vi "Line Configuration Dialog.vi"(8 "error in":errorcluster, 9 "engine configuration in":refnum<class "engine configuration.lvclass">, 10 "dds configuration":refnum<class "dds configuration.lvclass">, 11 "Line":T5) -> (0 "error out":errorcluster, 1 "success":bool, 2 "changed":bool, 3 "Mappings out":T4)   [LabVIEW 2020, in "DDS editor node.lvclass"]
uses:
  dds editor node.lvclass
  module/configuration/Line.ctl
  <vilib>/NI/Tag Bus Module Framework/channel/TBM channel.lvclass
  C:/Program Files (x86)/National Instruments/LabVIEW 2020/vi.lib/NI/Tag Bus/tag/tag descriptor.lvclass
  <vilib>/RTI DDS Toolkit/Types/RTI DDS Advanced Reader Configuration.ctl
  Mappings.ctl
  Map.ctl
  permissions.ctl
  <vilib>/NI/Module Execution Interface/Engine Configuration/engine configuration.lvclass
  module/configuration/dds configuration.lvclass
  C:/Program Files (x86)/National Instruments/LabVIEW 2020/vi.lib/NI/Configuration Framework/serializable configuration/NISE_CEF_serializable configuration.lvclass
  <vilib>/NI/Tag Bus Module Framework/channel/TBM channel.lvclass/TBM channel.ctl
  <vilib>/NI/Tag Bus/tag/tag descriptor.lvclass/tag descriptor.ctl
  <vilib>/NI/Configuration Framework/serializable configuration/NISE_CEF_serializable configuration.lvclass/NISE_CEF_serializable configuration.ctl
  <vilib>/NI/Tag Bus/tag/write tag name.vi
  <vilib>/NI/Tag Bus/tag/write data type.vi
  <vilib>/NI/Tag Bus Module Framework/channel/Write channel classification.vi
  <vilib>/NI/Tag Bus Module Framework/channel/Read channel classification.vi
  <vilib>/NI/Tag Bus/tag/read data type.vi
  <vilib>/NI/Configuration Framework/serializable configuration/Read UID.vi
  <vilib>/Utility/LVClass/Get LV Class Name.vi
  <vilib>/NI/Configuration Framework/error generator/NISE_error generator.vi
  <vilib>/NI/Tag Bus/tag/tag descriptor.lvclass
  <vilib>/RTI DDS Toolkit/Library/LVDDS_library.lvlib
panel:
  in  "Reader Configuration":T1={"typeName"="", "keyName"="", "domainParticipantQoSProfile"="", "dataReaderQoSProfile"="LabVIEWLibrary::DefaultProfile", "forceArrayMapping?"=FALSE, "forceExclusiveReader?"=FALSE, "forceRead? (only ExclusiveReader)"=FALSE, "forceUnboundedString?"=FALSE}
  in  "Domain ID":u32
  in  "Writer Configuration":T2={"typeName"="", "keyName"="", "domainParticipantQoSProfile"="", "dataWriterQoSProfile"="LabVIEWLibrary::DefaultProfile", "forceArrayMapping?"=FALSE, "forceUnboundedString?"=FALSE}
  out "errors":string
  in  "Access Type":T3
  in  "Mapped Tag":i32(listbox)
  in  "Data Type":i32(listbox)
  in  "Topic Name":string
  in  "cancel":bool
  in  "ok":bool
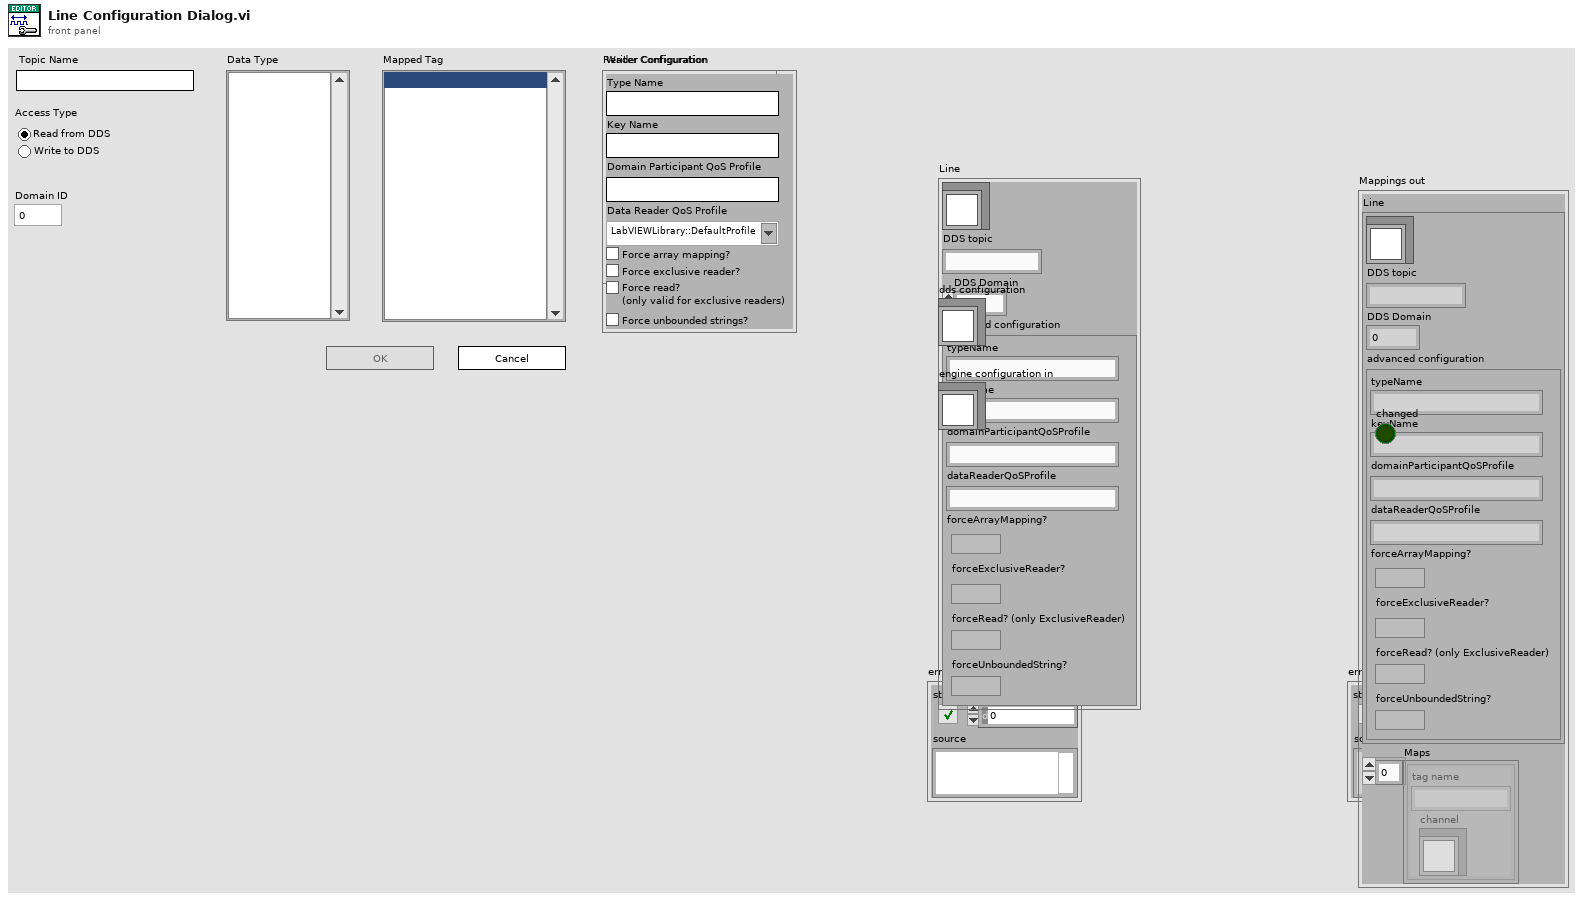
[diagram p1: front panel]
types:
  T1 = cluster{"typeName":string, "keyName":string, "domainParticipantQoSProfile":string, "dataReaderQoSProfile":string, "forceArrayMapping?":bool, "forceExclusiveReader?":bool, "forceRead? (only ExclusiveReader)":bool, "forceUnboundedString?":bool}
  T2 = cluster{"typeName":string, "keyName":string, "domainParticipantQoSProfile":string, "dataWriterQoSProfile":string, "forceArrayMapping?":bool, "forceUnboundedString?":bool}
  T3 = typedef "DDS editor node.lvclass/permissions.ctl" = enum32{"Read from DDS", "Write to DDS"}
  T4 = typedef "DDS editor node.lvclass/Mappings.ctl" = cluster{"Line":T5, "Maps":T7[]}
  T5 = typedef "DDS configuration.lvclass/Line.ctl" = cluster{"channel":refnum<class "TBM channel.lvclass">, "DDS topic":string, "DDS Domain":u32, "advanced configuration":T6}
  T6 = typedef "LVDDS_library.lvlib/RTI DDS Advanced Reader Configuration.ctl" = cluster{"typeName":string, "keyName":string, "domainParticipantQoSProfile":string, "dataReaderQoSProfile":string, "forceArrayMapping?":bool, "forceExclusiveReader?":bool, "forceRead? (only ExclusiveReader)":bool, "forceUnboundedString?":bool}
  T7 = typedef "DDS editor node.lvclass/Map.ctl" = cluster{"channel":refnum<class "TBM channel.lvclass">, "tag name":string}
  T8 = typedef "tag bus.lvlib/tag descriptor.lvclass/Data Type.ctl" = enum16{"Double", "Single", "I64", "I32", "I16", "I8", "U64", "U32", "U16", "U8", "Boolean", "String", "Array of Double", "Array of Single", "Array of I64", "Array of I32", "Array of I16", "Array of I8", "Array of U64", "Array of U32", "Array of U16", "Array of U8", "Array of Boolean", "Array of String"}
  T9 = typedef "TBM channel.lvclass/channel classification.ctl" = enum16{"input data", "output data", "processing parameter", "processing result"}
  T10 = typedef "LVDDS_library.lvlib/RTI DDS Advanced Writer Configuration.ctl" = cluster{"typeName":string, "keyName":string, "domainParticipantQoSProfile":string, "dataWriterQoSProfile":string, "forceArrayMapping?":bool, "forceUnboundedString?":bool}
  T11 = enum8{"Enabled", "Disabled", "Disabled and Grayed Out"}
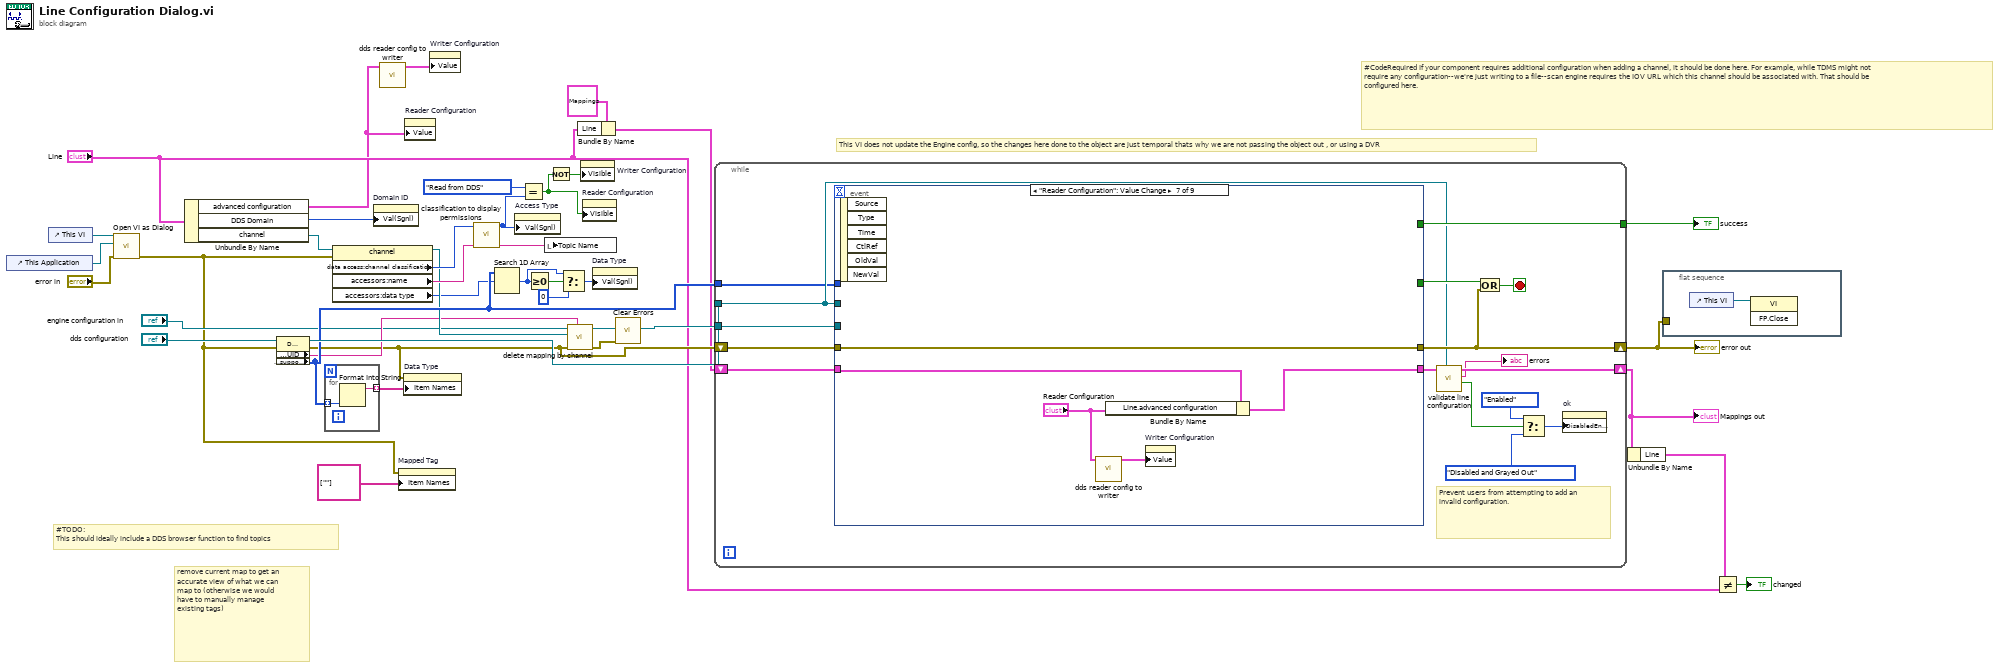
[diagram p0: block diagram]
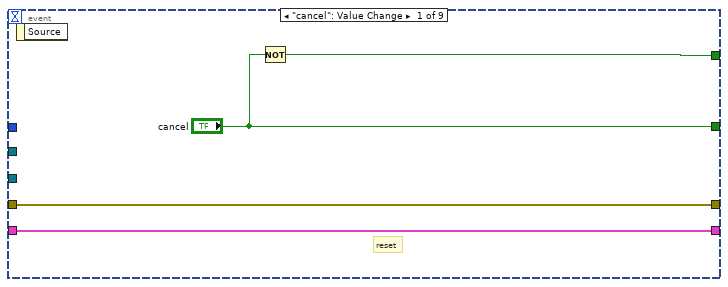
[diagram p2: hidden frame]
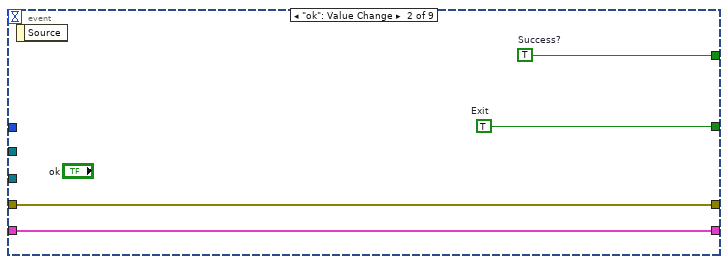
[diagram p3: hidden frame]
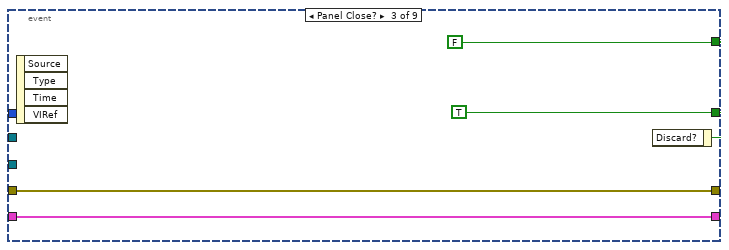
[diagram p4: hidden frame]
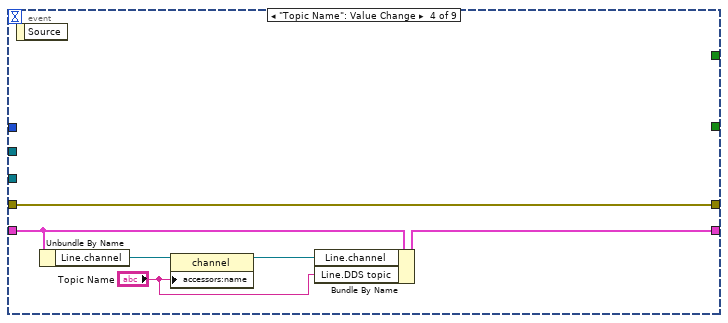
[diagram p5: hidden frame]
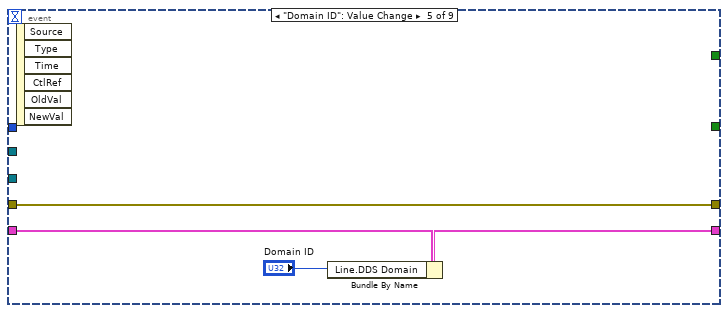
[diagram p6: hidden frame]
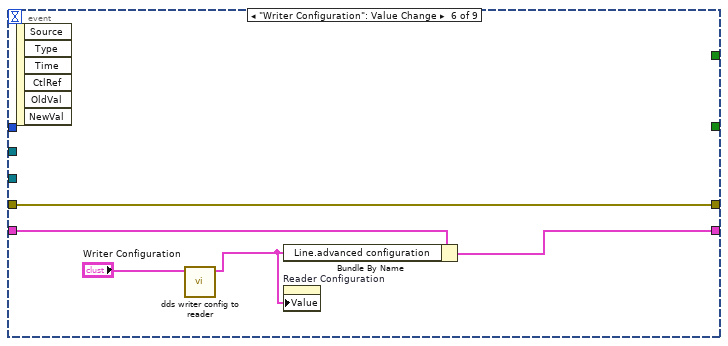
[diagram p7: hidden frame]
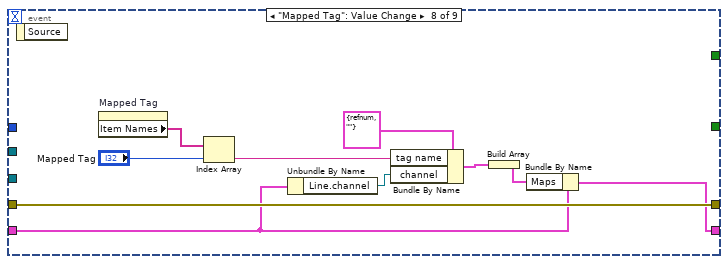
[diagram p8: hidden frame]
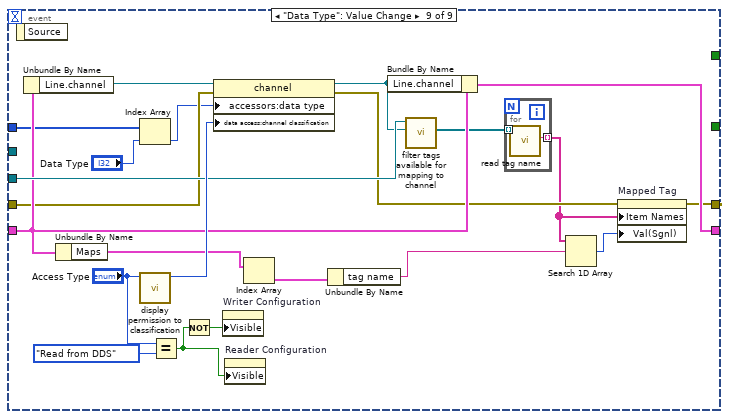
[diagram p9: hidden frame]
diagram:
  # "#TODO:\nThis should ideally include a DDS browser function to find topics"
  # "This VI does not update the Engine config, so the changes here done to the object are just temporal thats why we are not passing the object out , or using a DVR"
  # "remove current map to get an accurate view of what we can map to (otherwise we would have to manually manage existing tags)"
  # "#CodeRequired If your component requires additional configuration when adding a channel, it should be done here. For example, while TDMS might not require any configuration--we're just writing to a file--scan engine requires the IOV URL which this channel should be associated with. That should be configured here."
  n1 = control-ref of="This Application"() -> (w33:refnum<vi>)
  n2 = control-ref of="This VI"() -> (w32:refnum<vi>)
  n3 = call "Open VI as Dialog.vi"("error in (no error)"="error in", "This Application"=w33, "VI in"=w32) -> ("error out"=w13:errorcluster)  [unwired: 8 in]
  n4 = Unbundle By Name("Line") -> ("advanced configuration"=w2:T6, "DDS Domain"=w3:u32, "channel"=w28:refnum<class "TBM channel.lvclass">)
  n5 = property class="DDS module configuration"(reference="dds configuration", error in=w13) -> (reference out=w35:refnum<class "dds configuration.lvclass">, error out=w15:errorcluster, "Properties:UID"=w26:string, "Customize:Properties:supported types"=w34:T8[])
  n6 = for {
    tunnel: w34 -> [w40] mode=indexing
    tunnel: [w39] -> w25 mode=indexing
    n7 = Format Into String(w40) -> (resulting string=w39:string)  [unwired: 3 in, 1 out]
  }
  n8 = property class="channel"(reference=w28, error in=w13) -> (reference out=w27:refnum<class "TBM channel.lvclass">, "data access:channel classification"=w30:T9, "accessors:name"=w29:string, "accessors:data type"=w19:T8)  [unwired: 1 out]
  n9 = property on="Domain ID" class="DigNum (strict)"("Val(Sgnl)"=w3) -> ()  [unwired: 2 in, 2 out]
  n10 = call "dds reader config to writer.vi"("reader configuration"=w2) -> ("writer configuration"=w1:T10)  [unwired: 10 in]
  n11 = property on="Mapped Tag" class="LstBox (strict)"(error in=w13, "Item Names"=string[] [""]) -> ()  [unwired: 1 in, 2 out]
  n12 = property on="Data Type" class="LstBox (strict)"(error in=w15, "Item Names"=w25) -> ()  [unwired: 1 in, 2 out]
  n13 = property on="Reader Configuration" class="Clust (strict)"("Value"=w2) -> ()  [unwired: 2 in, 2 out]
  n14 = property on="Writer Configuration" class="Clust (strict)"("Value"=w1) -> ()  [unwired: 2 in, 2 out]
  n15 = call "classification to display permissions.vi"("channel classification"=w30) -> ("permissions"=w5:T3)  [unwired: 10 in]
  n16 = Search 1D Array(1D array=w34, element=w19) -> (index of element=w23:i32)  [unwired: 1 in]
  n17 = property on="Access Type" class="RadioBtnsControl (strict)"("Val(Sgnl)"=w5) -> ()  [unwired: 2 in, 2 out]
  n18 = Equal?(x=permissions."Read from DDS", y=w5) -> (x = y?=w7:bool)
  n19 = Greater Or Equal To 0?(x=w23) -> (x >= 0?=w24:bool)
  n20 = local write "Topic Name"(w29) -> ()
  n21 = Not(x=w7) -> (.not. x?=w6:bool)
  n22 = Select(t=w23, s=w24, f=0) -> (s? t:f=w21:i32)
  n23 = call <vilib>:"delete mapping by channel.vi"("owner ID"=w26, "error in"=w15, "channel"=w27, "engine configuration in"="engine configuration in") -> ("error out"=w18:errorcluster, "engine configuration out"=w36:refnum<class "engine configuration.lvclass">)  [unwired: 6 in]
  n24 = Bundle By Name(cluster=T4 {"Line"={"channel"=refnum, "DDS topic"="", "DDS Domain"=0, "advanced configuration"={"typeName"="", "keyName"="", "domainParticipantQoSProfile"="", "dataReaderQoSProfile"="", "forceArrayMapping?"=FALSE, "forceExclusiveReader?"=FALSE, "forceRead? (only ExclusiveReader)"=FALSE, "forceUnboundedString?"=FALSE}}, "Maps"=[]} ("Mappings out"), "Line"="Line") -> (w10:T4)
  n25 = property on="Writer Configuration" class="Clust (strict)"("Visible"=w6) -> ()  [unwired: 2 in, 2 out]
  n26 = property on="Reader Configuration" class="Clust (strict)"("Visible"=w7) -> ()  [unwired: 2 in, 2 out]
  n27 = property on="Data Type" class="LstBox (strict)"("Val(Sgnl)"=w21) -> ()  [unwired: 2 in, 2 out]
  n28 = call <vilib>:"Clear Errors.vi"("error in (no error)"=w18) -> ()  [unwired: 5 in, 2 out]
  n29 = while {
    shift-right: [w48] -> w31
    shift-left: w15 -> [w55]
    tunnel: [w54] -> w38
    shift-right: [w49] -> w8
    shift-left: w10 -> [w51]
    tunnel: w36 -> [w56]
    tunnel: w35 -> [w43]
    tunnel: w34 -> [w42]
    stop <- w52 stop-if-true
    # "Prevent users from attempting to add an invalid configuration."
    n30 = event shown="[6] \"Reader Configuration\": Value Change" {
      selector: _ -> [_ _ _ _ _ _ _ _ _]
      dyn-events: _ -> [_ _ _ _ _ _ _ _ _]
      timeout: _ -> [_ _ _ _ _ _ _ _ _]
      tunnel: w56 -> [_ _ _ _ _ _ _ _ w118]
      tunnel: w55 -> [w60 w64 w68 w74 w78 w83 w88 w98 w113]
      tunnel: [w60 w64 w68 w74 w78 w83 w88 w98 w108] -> w48
      tunnel: [w59 w61 FALSE _ _ _ _ _ _] -> w54
      tunnel: ["cancel" w62 w66 _ _ _ _ _ _] -> w53
      tunnel: w51 -> [w57 w63 w65 w72 w77 w81 w87 w92 w116]
      tunnel: [w57 w63 w65 w73 w76 w80 w86 w89 w115] -> w50
      tunnel: w43 -> [_ _ _ _ _ _ _ _ _]
      tunnel: w42 -> [_ _ _ _ _ _ _ _ w112]
      event "cancel": Value Change {
        # "reset"
        n31 = event-data() -> ()  [unwired: 1 in, 1 out]
        n32 = Not(x="cancel") -> (.not. x?=w59:bool)
      }
      event "ok": Value Change {
        w61 = TRUE  # Success?
        w62 = TRUE  # Exit
        n33 = event-data() -> ()  [unwired: 1 in, 1 out]
      }
      event Panel Close? {
        w66 = TRUE ("cancel")
        n34 = event-data() -> ()  [unwired: 1 in, 4 out]
        n35 = event-data("Discard?"=w66) -> ()  [unwired: 1 in, 1 out]
      }
      event "Topic Name": Value Change {
        n36 = event-data() -> ()  [unwired: 1 in, 1 out]
        n37 = Unbundle By Name(w72) -> ("Line.channel"=w71:refnum<class "TBM channel.lvclass">)
        n38 = property class="channel"(reference=w71, "accessors:name"="Topic Name") -> (reference out=w70:refnum<class "TBM channel.lvclass">)  [unwired: 1 in, 1 out]
        n39 = Bundle By Name(cluster=w72, "Line.channel"=w70, "Line.DDS topic"="Topic Name") -> (w73:T4)
      }
      event "Domain ID": Value Change {
        n40 = event-data() -> ()  [unwired: 1 in, 6 out]
        n41 = Bundle By Name(cluster=w77, "Line.DDS Domain"="Domain ID") -> (w76:T4)
      }
      event "Writer Configuration": Value Change {
        n42 = event-data() -> ()  [unwired: 1 in, 6 out]
        n43 = call "dds writer config to reader.vi"("writer configuration"="Writer Configuration") -> ("reader configuration"=w79:T6)  [unwired: 10 in]
        n44 = Bundle By Name(cluster=w81, "Line.advanced configuration"=w79) -> (w80:T4)
        n45 = property on="Reader Configuration" class="Clust (strict)"("Value"=w79) -> ()  [unwired: 2 in, 2 out]
      }
      event "Reader Configuration": Value Change {
        n46 = event-data() -> ()  [unwired: 1 in, 6 out]
        n47 = call "dds reader config to writer.vi"("reader configuration"="Reader Configuration") -> ("writer configuration"=w85:T10)  [unwired: 10 in]
        n48 = Bundle By Name(cluster=w87, "Line.advanced configuration"="Reader Configuration") -> (w86:T4)
        n49 = property on="Writer Configuration" class="Clust (strict)"("Value"=w85) -> ()  [unwired: 2 in, 2 out]
      }
      event "Mapped Tag": Value Change {
        n50 = event-data() -> ()  [unwired: 1 in, 1 out]
        n51 = property on="Mapped Tag" class="LstBox (strict)"() -> ("Item Names"=w96:string[])  [unwired: 2 in, 2 out]
        n52 = Index Array(array=w96, index="Mapped Tag") -> (element=w95:string)
        n53 = Unbundle By Name(w92) -> ("Line.channel"=w93:refnum<class "TBM channel.lvclass">)
        n54 = Bundle By Name(cluster=T7 {"channel"=refnum, "tag name"=""} ("Map"), "tag name"=w95, "channel"=w93) -> (w91:T7)
        n55 = Build Array(w91) -> (w90:T7[])
        n56 = Bundle By Name(cluster=w92, "Maps"=w90) -> (w89:T4)
      }
      event "Data Type": Value Change {
        n57 = event-data() -> ()  [unwired: 1 in, 1 out]
        n58 = Unbundle By Name(w116) -> ("Line.channel"=w120:refnum<class "TBM channel.lvclass">)
        n59 = Unbundle By Name(w116) -> ("Maps"=w105:T7[])
        n60 = Index Array(array=w112, index="Data Type") -> (element=w110:T8)
        n61 = call "display permission to classification.vi"("display permissions"="Access Type") -> ("channel classification"=w119:T9)  [unwired: 10 in]
        n62 = Equal?(x="Access Type", y=permissions."Read from DDS") -> (x = y?=w99:bool)
        n63 = Not(x=w99) -> (.not. x?=w100:bool)
        n64 = property class="channel"(reference=w120, error in=w113, "accessors:data type"=w110, "data access:channel classification"=w119) -> (reference out=w117:refnum<class "TBM channel.lvclass">, error out=w109:errorcluster)
        n65 = property on="Writer Configuration" class="Clust (strict)"("Visible"=w100) -> ()  [unwired: 2 in, 2 out]
        n66 = property on="Reader Configuration" class="Clust (strict)"("Visible"=w99) -> ()  [unwired: 2 in, 2 out]
        n67 = Index Array(array=w105) -> (element=w104:T7)  [unwired: 1 in]
        n68 = Unbundle By Name(w104) -> ("tag name"=w103:string)
        n69 = Bundle By Name(cluster=w116, "Line.channel"=w117) -> (w115:T4)
        n70 = call-dynamic "filter tags available for mapping to channel.vi"("channel to map to"=w117, "engine configuration in"=w118) -> ("filtered tags"=w114:refnum<class "tag descriptor.lvclass">[])  [unwired: 8 in, 1 out]
        n71 = for {
          tunnel: w114 -> [w122] mode=indexing
          tunnel: [w121] -> w107 mode=indexing
          n72 = call <vilib>:"read tag name.vi"("system tag in"=w122) -> ("name"=w121:string)  [unwired: 8 in, 2 out]
        }
        n73 = Search 1D Array(1D array=w107, element=w103) -> (index of element=w106:i32)  [unwired: 1 in]
        n74 = property on="Mapped Tag" class="LstBox (strict)"(error in=w109, "Item Names"=w107, "Val(Sgnl)"=w106) -> (error out=w108:errorcluster)  [unwired: 1 in, 1 out]
      }
    }
    n75 = call "validate line configuration.vi"("module"=w43, "Mappings in"=w50) -> ("valid?"=w47:bool, "errors"=→"errors":string, "Mappings out"=w49:T4)  [unwired: 7 in]
    n76 = Compound Arithmetic op=OR(w53, w48) -> (w52:bool)
    n77 = Select(t=T11."Enabled" ("Disabled"), s=w47, f=T11."Disabled and Grayed Out") -> (s? t:f=w44:T11)
    n78 = property on="ok" class="Bool"("DisabledEnum"=w44) -> ()  [unwired: 2 in, 2 out]
  }
  "error out" <- w31
  "success" <- w38
  "Mappings out" <- w8
  n79 = Unbundle By Name(w8) -> ("Line"=w9:T5)
  n80 = flat-sequence {
    tunnel: w31 -> [_]
    frame #0 {
      n81 = control-ref of="This VI"() -> (w123:refnum<vi>)
      n82 = invoke class="VI" method="FP.Close"(reference=w123) -> ()  [unwired: 2 in, 3 out]
    }
  }
  n83 = Not Equal?(x=w9, y="Line") -> (x != y?=→"changed":bool)
